vi "Read Depends.vi"(8 "error in":errorcluster, 11 "Custom Device reference in":refnum<k24>) -> (0 "error out":errorcluster caption="error in", 2 "Dependencies":T3(array[cluster]), 3 "Custom Device reference out":refnum<k24>)   [LabVIEW 2015, in "Configuration Tool.lvlib"]
uses:
  Configuration Tool.lvlib
  NationalInstruments.VeriStand.XMLReader
  XML Controls/Target.ctl
  XML Controls/Path Cluster.ctl
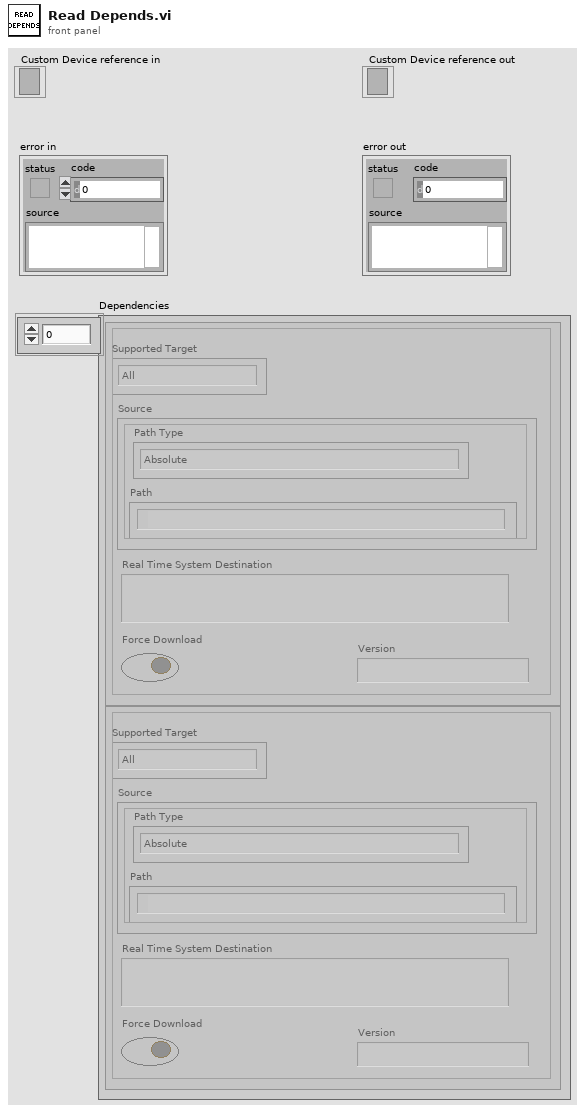
[diagram p1: front panel]
types:
  T1 = typedef "Configuration Tool.lvlib/Target.ctl" = enum16{"All", "Pharlap", "VxWorks", "Windows", "Linux_32_ARM", "Linux_x64", "PharlapWindows", "PharlapVxWorks", "VxWorksWindows"}
  T2 = typedef "Configuration Tool.lvlib/Path Cluster.ctl" = cluster{"Path":path, "Path Type":enum16{"Absolute", "To Base", "To Common Doc Dir", "To Application Data Dir"}}
  T3 = cluster{"Supported Target":T1, "Source":T2, "Real Time System Destination":string, "Force Download":bool, "Version":string}[]
  T4 = cluster{"Supported Target":T1, "Source":T2, "Real Time System Destination":string, "Force Download":bool, "Version":string}
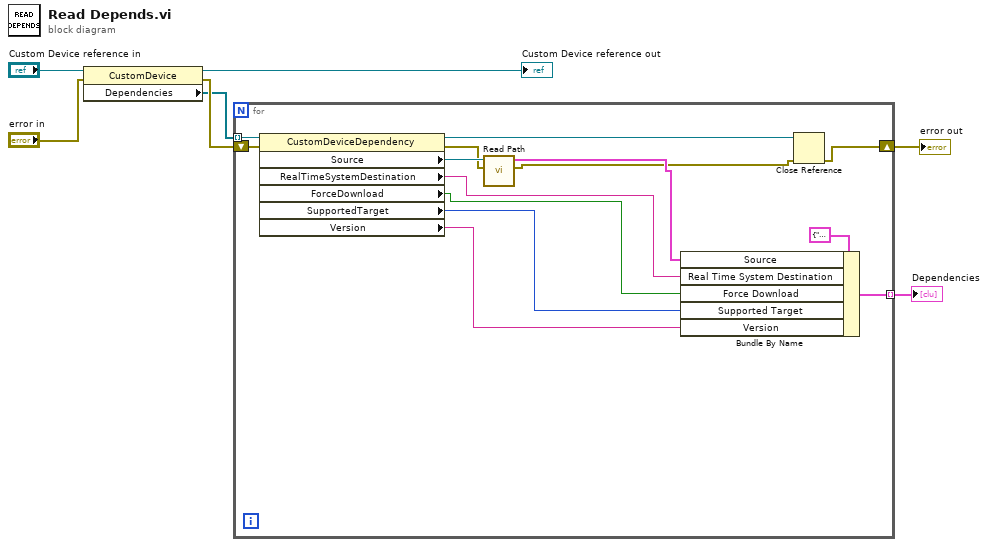
[diagram p0: block diagram]
diagram:
  n1 = property class="CustomDevice"(reference="Custom Device reference in", error in="error in") -> (reference out=→"Custom Device reference out":refnum<k24>, error out=w4:errorcluster, "Dependencies"=w3:refnum<k24>[])
  n2 = for {
    tunnel: w3 -> [w20] mode=indexing
    shift-right: [w13] -> w1
    shift-left: w4 -> [w21]
    tunnel: [w12] -> w2 mode=indexing
    n3 = property class="CustomDeviceDependency"(reference=w20, error in=w21) -> (reference out=w18:refnum<k24>, error out=w10:errorcluster, "Source"=w17:refnum<k24>, "RealTimeSystemDestination"=w14:string, "ForceDownload"=w15:bool, "SupportedTarget"=w11:i32, "Version"=w16:string)
    n4 = call "Read Path.vi"("Error In"=w10, "Path .NET Ref"=w17) -> ("Error Out"=w8:errorcluster, "Path Properties"=w9:T2)  [unwired: 8 in]
    n5 = Bundle By Name(cluster=T4 {"Supported Target"=enum."All", "Source"={"Path"=path "", "Path Type"=enum."Absolute"}, "Real Time System Destination"="", "Force Download"=FALSE, "Version"=""} ("Dependency"), "Source"=w9, "Real Time System Destination"=w14, "Force Download"=w15, "Supported Target"=w11, "Version"=w16) -> (w12:T4)
    n6 = Close Reference(reference=w18, error in (no error)=w8) -> (error out=w13:errorcluster)
  }
  "error out" <- w1
  "Dependencies" <- w2
